vi "testingvi.vi"() -> ()   [LabVIEW 2011, in "Hardware.lvlib" / "Channels.lvlib" / "niDAQmxAO.lvclass"]
uses:
  niDAQmxAO.lvclass
  <vilib>/DAQmx/write.llb/DAQmx Write (Analog 1D Wfm NChan NSamp).vi
  <vilib>/DAQmx/create/channels.llb/DAQmx Create Channel (AO-Voltage-Basic).vi
  <vilib>/DAQmx/configure/timing.llb/DAQmx Timing (Sample Clock).vi
  <vilib>/DAQmx/configure/trigger.llb/DAQmx Start Trigger (Digital Edge).vi
  <vilib>/DAQmx/miscellaneous.llb/DAQmx Fill In Error Info.vi
  Program Files/National Instruments/LabVIEW 2011/resource/objmgr/daqmx.rc
  <vilib>/measure/NI_MABase.lvlib
panel:
  out "String 2":string
  out "String":string
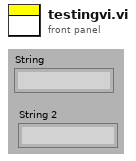
[diagram p1: front panel]
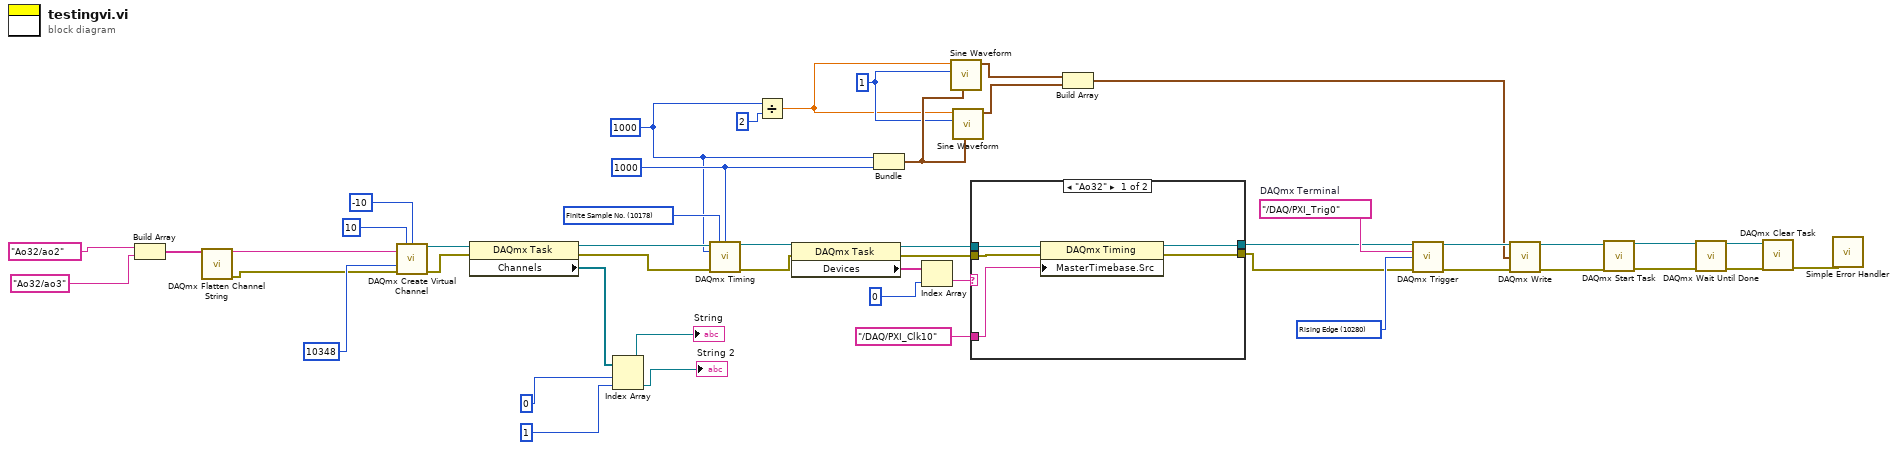
[diagram p0: block diagram]
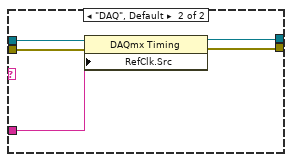
[diagram p2: hidden frame]
diagram:
  w19 = 1
  w14 = tag "/DAQ/PXI_Trig0"  # DAQmx Terminal
  w29 = u16 10280 items=["Rising Edge"=10280]
  w18 = 1000
  w30 = u16 10178 items=["Finite Sample No."=10178]
  w15 = 1000
  n1 = Build Array("Ao32/ao2", "Ao32/ao3") -> (w40:string[])
  n2 = call <vilib>:"DAQmx Flatten Channel String.vi"("names in"=w40) -> ("names out"=w39:string, "error out"=w33:errorcluster)  [unwired: 13 in]
  n3 = call-poly <vilib>:"DAQmx Create Virtual Channel.vi"("maximum value"=10, "minimum value"=-10, "physical channels"=w39, "units"=10348, "error in"=w33) -> ("task out"=w45:refnum<k21>, "error out"=w44:errorcluster)  [unwired: 9 in]
  n4 = property class="DAQmx Task"(reference=w45, error in=w44) -> (reference out=w32:refnum<k21>, error out=w31:errorcluster, "Channels"=w38:refnum<k21>[])
  n5 = Index Array(array=w38, index #1=0, index #2=1) -> (element #1=→"String":refnum<k21>, element #2=→"String 2":refnum<k21>)
  n6 = call-poly <vilib>:"DAQmx Timing.vi"("task/channels in"=w32, "sample mode"=w30, "samples per channel"=w18, "rate"=w15, "error in"=w31) -> ("task out"=w13:refnum<k21>, "error out"=w12:errorcluster)  [unwired: 9 in]
  n7 = Divide(x=w15, y=2) -> (x/y=w17:dbl)
  n8 = property class="DAQmx Task"(reference=w13, error in=w12) -> (reference out=w11:refnum<k21>, error out=w10:errorcluster, "Devices"=w7:tag[])
  n9 = Bundle(w15, w18) -> (w20:cluster{i32, i32})  [unwired: 1 in]
  n10 = Index Array(array=w7, index=0) -> (element=w6:tag)
  n11 = call <vilib>:"Sine Waveform.vi"("sampling info"=w20, "amplitude"=w19, "frequency"=w17) -> ("signal out"=w3:waveform(dbl))  [unwired: 7 in, 1 out]
  n12 = call <vilib>:"Sine Waveform.vi"("sampling info"=w20, "amplitude"=w19, "frequency"=w17) -> ("signal out"=w2:waveform(dbl))  [unwired: 7 in, 1 out]
  n13 = case shown="\"Ao32\"" w6 {
    tunnel: w11 -> [w53 w58]
    tunnel: w10 -> [w52 w57]
    tunnel: [w50 w56] -> w9
    tunnel: [w49 w55] -> w8
    tunnel: "/DAQ/PXI_Clk10" -> [w51 w54]
    frame "Ao32" {
      n14 = property class="DAQmx Timing"(reference=w53, error in=w52, "MasterTimebase.Src"=w51) -> (reference out=w50:refnum<k21>, error out=w49:errorcluster)
    }
    frame "DAQ", Default {
      n15 = property class="DAQmx Timing"(reference=w58, error in=w57, "RefClk.Src"=w54) -> (reference out=w56:refnum<k21>, error out=w55:errorcluster)
    }
  }
  n16 = Build Array(w3, w2) -> (w1:waveform(dbl)[])
  n17 = call-poly <vilib>:"DAQmx Trigger.vi"("task/channels in"=w9, "source"=w14, "edge"=w29, "error in"=w8) -> ("task out"=w28:refnum<k21>, "error out"=w27:errorcluster)  [unwired: 10 in]
  n18 = call-poly <vilib>:"DAQmx Write.vi"("task/channels in"=w28, "data"=w1, "error in"=w27) -> ("task out"=w26:refnum<k21>, "error out"=w25:errorcluster)  [unwired: 10 in, 1 out]
  n19 = call <vilib>:"DAQmx Start Task.vi"("task/channels in"=w26, "error in"=w25) -> ("task out"=w24:refnum<k21>, "error out"=w23:errorcluster)  [unwired: 12 in]
  n20 = call <vilib>:"DAQmx Wait Until Done.vi"("task/channels in"=w24, "error in"=w23) -> ("task out"=w21:refnum<k21>, "error out"=w22:errorcluster)  [unwired: 12 in]
  n21 = call <vilib>:"DAQmx Clear Task.vi"("task in"=w21, "error in"=w22) -> ("error out"=w43:errorcluster)  [unwired: 13 in]
  n22 = call <vilib>:"Simple Error Handler.vi"("error in (no error)"=w43) -> ()  [unwired: 4 in, 5 out]
